vi "Update UI per Reference.vi"(8 "error in (no error)":errorcluster, 11 "Analyze Results Fluence in":refnum<class "Analyze Results Fluence.lvclass">) -> (0 "error out":errorcluster, 3 "Analyze Results Fluence out":refnum<class "Analyze Results Fluence.lvclass">)   [LabVIEW 2014, in "Analyze Results Fluence.lvclass"]
uses:
  Analyze Results Fluence.lvclass
  Analyze Results Fluence.lvclass/Analyze Results Fluence.ctl
  Results Base/Analyze Results Base.lvclass
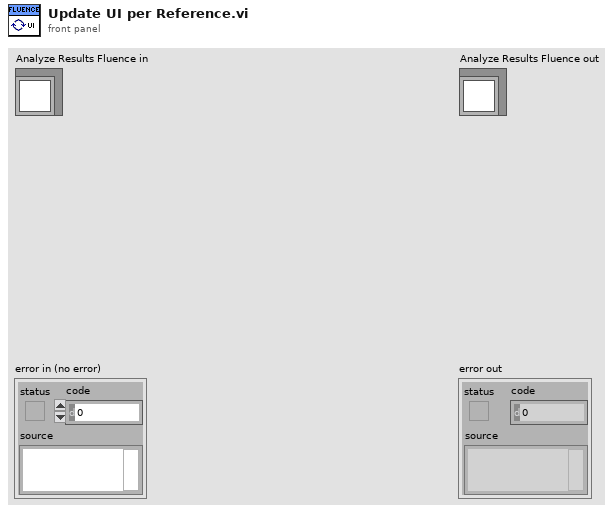
[diagram p1: front panel]
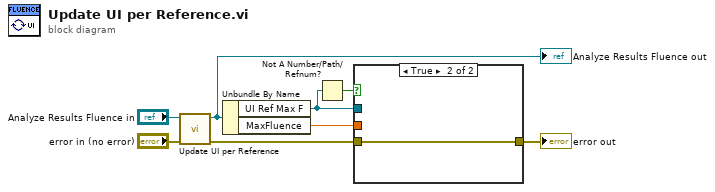
[diagram p0: block diagram]
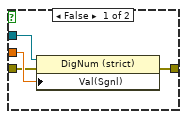
[diagram p2: hidden frame]
diagram:
  n1 = call-parent "Update UI per Reference.vi"("error in (no error)"="error in (no error)", "Analyze Results Base in"="Analyze Results Fluence in") -> ("error out"=w2:errorcluster, "Analyze Results Base out"=w6:refnum<class "Analyze Results Fluence.lvclass">)  [unwired: 8 in]
  "Analyze Results Fluence out" <- w6
  n2 = Unbundle By Name(w6) -> ("UI Ref Max F"=w4:refnum<vi>, "MaxFluence"=w3:dbl[unit])
  n3 = Not A Number/Path/Refnum?(number/path/refnum=w4) -> (NaN/Path/Refnum?=w5:bool)
  n4 = case shown="True" w5 {
    tunnel: w4 -> [w12 _]
    tunnel: w3 -> [w11 _]
    tunnel: w2 -> [w10 w13]
    tunnel: [w9 w13] -> w1
    frame False {
      n5 = property class="DigNum (strict)"(reference=w12, error in=w10, "Val(Sgnl)"=w11) -> (error out=w9:errorcluster)  [unwired: 1 out]
    }
    frame True {
    }
  }
  "error out" <- w1
